vi "Update Boolean Value.vi"(9 "Value":bool, 10 "Tree Tag":string, 11 "Settings In":T1) -> (3 "Settings Out":T1)   [LabVIEW 2024, in "Sequencer with Output Values.lvlib" / "Sequencer with Output Values.lvclass"]
uses:
  Sequencer with Output Values.lvclass
  Params.ctl
  Step Settings.ctl
  Global Tree Data.vi
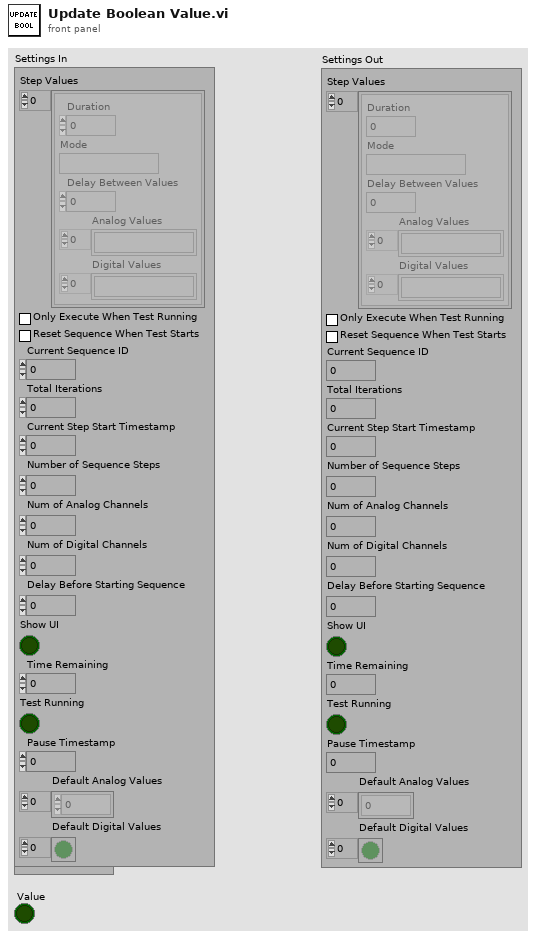
[diagram p1: front panel]
types:
  T1 = typedef "Sequencer with Output Values.lvlib/Sequencer with Output Values.lvclass/Params.ctl" = cluster{"Step Values":T2[], "Only Execute When Test Running":bool, "Reset Sequence When Test Starts":bool, "Current Sequence ID":u32, "Total Iterations":u32, "Current Step Start Timestamp":dbl, "Number of Sequence Steps":i32, "Num of Analog Channels":i32, "Num of Digital Channels":i32, "Delay Before Starting Sequence":dbl, "Show UI":bool, "Time Remaining":dbl, "Test Running":bool, "Pause Timestamp":dbl, "Default Analog Values":dbl[], "Default Digital Values":bool[]}
  T2 = typedef "Sequencer with Output Values.lvlib/Sequencer with Output Values.lvclass/Step Settings.ctl" = cluster{"Duration":dbl, "Mode":string, "Delay Between Values":dbl, "Analog Values":string[], "Digital Values":string[]}
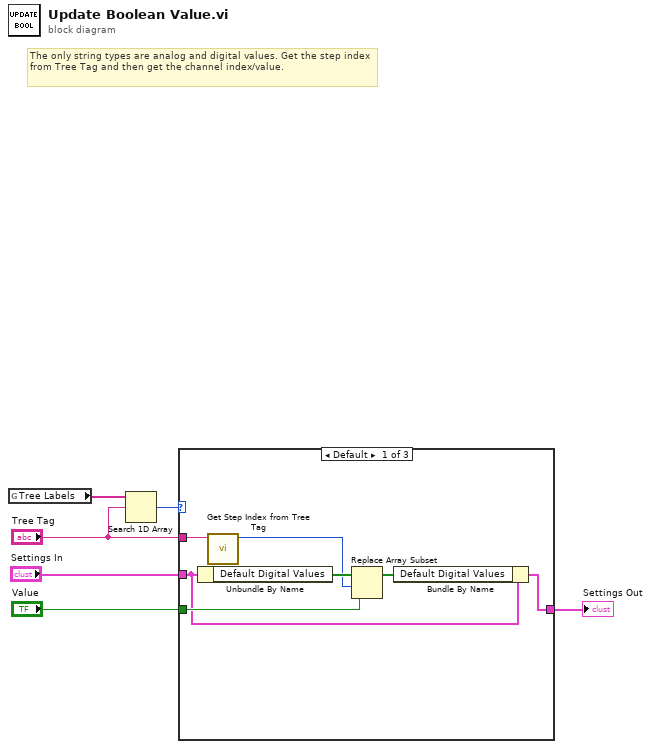
[diagram p0: block diagram]
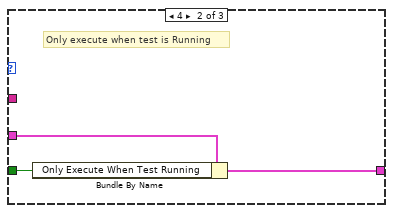
[diagram p2: hidden frame]
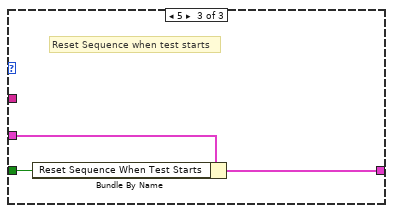
[diagram p3: hidden frame]
diagram:
  # "The only string types are analog and digital values. Get the step index from Tree Tag and then get the channel index/value."
  n1 = global read "Global Tree Data.vi" "Tree Labels"() -> (w6:string[])
  n2 = Search 1D Array(1D array=w6, element="Tree Tag") -> (index of element=w5:i32)  [unwired: 1 in]
  n3 = case shown="Default" w5 {
    tunnel: "Settings In" -> [w9 w16 w19]
    tunnel: "Value" -> [w10 w15 w18]
    tunnel: [w7 w14 w17] -> w2
    tunnel: "Tree Tag" -> [w13 _ _]
    frame Default {
      n4 = Unbundle By Name(w9) -> ("Default Digital Values"=w12:bool[])
      n5 = call "Get Step Index from Tree Tag.vi"("Tree Tag"=w13) -> ("Step Index"=w11:i32)  [unwired: 9 in, 1 out]
      n6 = Replace Array Subset(array=w12, new element=w10, index=w11) -> (w8:bool[])
      n7 = Bundle By Name(cluster=w9, "Default Digital Values"=w8) -> (w7:T1)
    }
    frame 4 {
      # "Only execute when test is Running"
      n8 = Bundle By Name(cluster=w16, "Only Execute When Test Running"=w15) -> (w14:T1)
    }
    frame 5 {
      # "Reset Sequence when test starts"
      n9 = Bundle By Name(cluster=w19, "Reset Sequence When Test Starts"=w18) -> (w17:T1)
    }
  }
  "Settings Out" <- w2
